vi "mqttCmdAcknowledge.vi"(0 "_mqtt in":refnum<class "mqttCmdSubscribe.lvclass">, 7 "mqtt in":refnum<class "mqtt.lvclass">, 11 "error in (no error)":errorcluster) -> (4 "_mqtt out":refnum<class "mqttCmdSubscribe.lvclass">, 8 "notification":T1, 15 "error out":errorcluster)   [LabVIEW 2014, in "labview-mqtt.lvlib" / "mqttCmdSubscribe.lvclass"]
uses:
  mqttCmdSubscribe.lvclass
  mqttTypedef/mqttRXdataCluster.ctl
  mqttTypedef/mqttFixedHeaderResponse.ctl
  mqttTypedef/mqttQOSlevel.ctl
  mqttTypedef/mqttMessageType.ctl
  mqtt.lvclass
  mqttCmd.lvclass/mqttCmd.ctl
  mqttCmdSubscribe.lvclass/mqttCmdSubscribe.ctl
  labview-mqtt.lvlib
  mqttCmd.lvclass
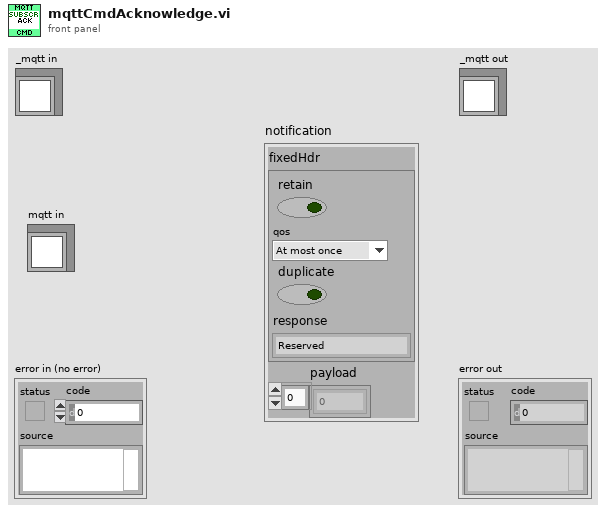
[diagram p1: front panel]
types:
  T1 = typedef "labview-mqtt.lvlib/mqttRXdataCluster.ctl" = cluster{"fixedHdr":T2, "payload":u8[]}
  T2 = typedef "labview-mqtt.lvlib/mqttFixedHeaderResponse.ctl" = cluster{"retain":bool, "qos":T3, "duplicate":bool, "response":T4}
  T3 = typedef "labview-mqtt.lvlib/mqttQOSlevel.ctl" = enum8{"At most once", "At least once", "Exactly once", "Reserved"}
  T4 = typedef "labview-mqtt.lvlib/mqttMessageType.ctl" = enum32{"Reserved", "CONNECT", "CONNACK", "PUBLISH", "PUBACK", "PUBREC", "PUBREL", "PUBCOMP", "SUBSCRIBE", "SUBACK", "UNSUBSCRIBE", "UNSUBACK", "PINGREQ", "PINGRESP", "DISCONNECT", "Reserved2"}
  T5 = typedef "labview-mqtt.lvlib/mqttSubscribeCluster.ctl" = cluster{"Topic":string, "QoS":T3}
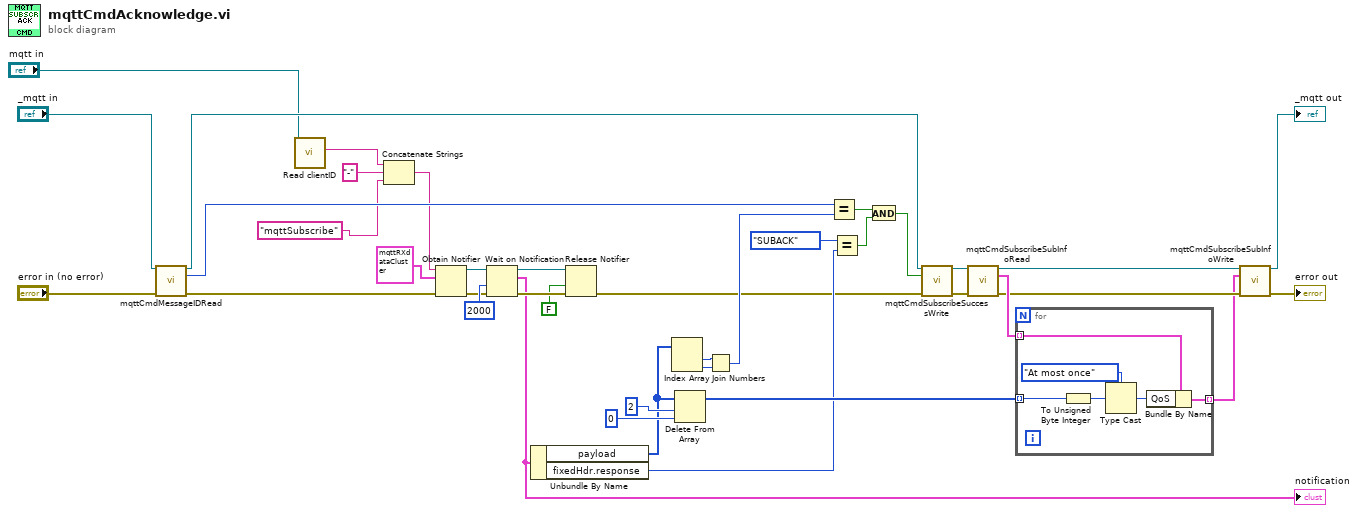
[diagram p0: block diagram]
diagram:
  n1 = call "mqttCmdMessageIDRead.vi"("mqttBrokerCommand in"="_mqtt in", "error in (no error)"="error in (no error)") -> ("mqttBrokerCommand out"=w18:refnum<class "mqttCmdSubscribe.lvclass">, "messageID"=w17:u16, "error out"=w20:errorcluster)  [unwired: 11 in]
  n2 = call-dynamic "Read clientID.vi"("mqtt in"="mqtt in") -> ("clientID"=w4:string)  [unwired: 8 in, 2 out]
  n3 = Concatenate Strings(w4, "-" ("string"), "mqttSubscribe" ("name (unnamed)")) -> (w1:string)
  n4 = Obtain Notifier(name (unnamed)=w1, notification data type=T1 {"fixedHdr"={"retain"=FALSE, "qos"=enum."At most once", "duplicate"=FALSE, "response"=enum."Reserved"}, "payload"=[]} ("notification"), error in (no error)=w20) -> (notifier out=w25:refnum<notifier>, error out=w23:errorcluster)  [unwired: 1 in, 1 out]
  n5 = Wait on Notification(notifier=w25, timeout in ms (-1)=2000, error in (no error)=w23) -> (notifier out=w31:refnum<notifier>, notification=w15:T1, error out=w30:errorcluster)  [unwired: 1 in, 1 out]
  "notification" <- w15
  n6 = Unbundle By Name(w15) -> ("payload"=w32:u8[], "fixedHdr.response"=w16:T4)
  n7 = Release Notifier(notifier=w31, force destroy? (F)=FALSE, error in (no error)=w30) -> (error out=w14:errorcluster)  [unwired: 2 out]
  n8 = Index Array(array=w32) -> (element #1=w28:u8, element #2=w27:u8)  [unwired: 2 in]
  n9 = Delete From Array(array=w32, length=2, index=0) -> (array with subset deleted=w39:u8[])  [unwired: 1 out]
  n10 = Join Numbers(hi=w28, lo=w27) -> ((hi.lo)=w38:u16)
  n11 = Equal?(x=w17, y=w38) -> (x = y?=w35:bool)
  n12 = Equal?(x=mqttMessageType."SUBACK", y=w16) -> (x = y?=w36:bool)
  n13 = And(x=w35, y=w36) -> (x .and. y?=w22:bool)
  n14 = call "mqttCmdSubscribeSuccessWrite.vi"("mqttBrokerCommand in"=w18, "success"=w22, "error in (no error)"=w14) -> ("mqttBrokerCommand out"=w12:refnum<class "mqttCmdSubscribe.lvclass">, "error out"=w13:errorcluster)  [unwired: 11 in]
  n15 = call "mqttCmdSubscribeSubInfoRead.vi"("mqttSubscribe in"=w12, "error in (no error)"=w13) -> ("mqttSubscribe out"=w8:refnum<class "mqttCmdSubscribe.lvclass">, "subscriptionInfo"=w11:T5[], "error out"=w10:errorcluster)  [unwired: 11 in]
  n16 = for {
    tunnel: w39 -> [w44] mode=indexing
    tunnel: w11 -> [w42] mode=indexing
    tunnel: [w40] -> w9 mode=indexing
    n17 = To Unsigned Byte Integer(number=w44) -> (unsigned 8bit integer=w45:u8)
    n18 = Type Cast(type=mqttQOSlevel."At most once" ("fixedHdr.qos"), x=w45) -> (*(type *) &x=w41:T3)
    n19 = Bundle By Name(cluster=w42, "QoS"=w41) -> (w40:T5)
  }
  n20 = call "mqttCmdSubscribeSubInfoWrite.vi"("mqttSubscribe in"=w8, "subscriptionInfo"=w9, "error in (no error)"=w10) -> ("mqttSubscribe out"=→"_mqtt out":refnum<class "mqttCmdSubscribe.lvclass">, "error out"=→"error out":errorcluster)  [unwired: 11 in]
